vi "TIO Stream Write.vi"(6 "Routing":string, 7 "error in (no error)":errorcluster, 8 "Type":T1(ring)=enum."RPC Request", 9 "Payload":string, 10 "TS Connection":T2={"Type"=enum."TCP", "Serial"="serial:///dev/cu.usbserial-00000", "TCP"=refnum, "Timeout"=500}) -> (0 "error out":errorcluster, 3 "TS Connection":T2={"Type"=enum."TCP", "Serial"="serial:///dev/cu.usbserial-00000", "TCP"=refnum, "Timeout"=500})   [LabVIEW 2016]
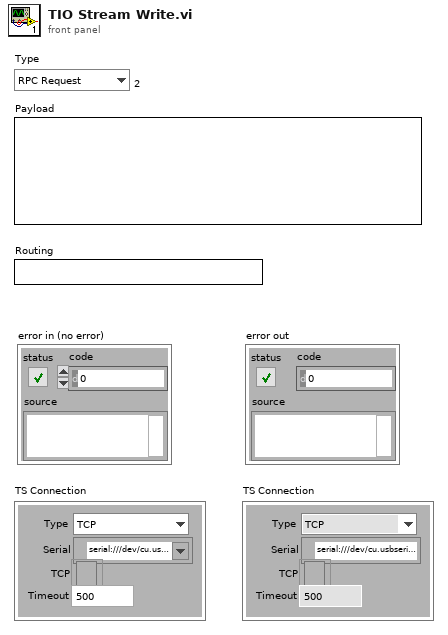
[diagram p1: front panel]
types:
  T1 = enum8{"Invalid", "Log", "RPC Request", "RPC Reply", "RPC Error", "Stream Description", "User"}
  T2 = cluster{"Type":enum16{"TCP", "Serial"}, "Serial":refnum<visa-resource-name>, "TCP":refnum<k5>, "Timeout":u32}
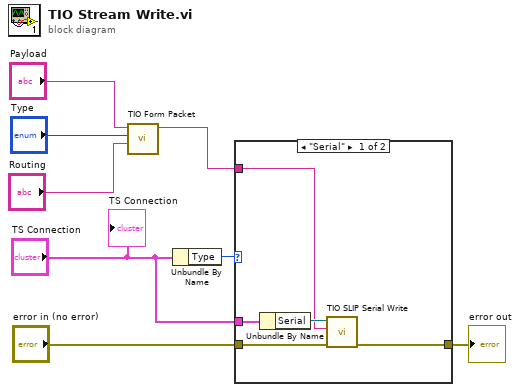
[diagram p0: block diagram]
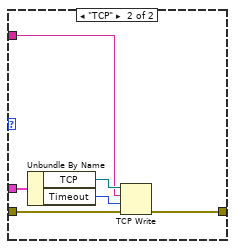
[diagram p2: hidden frame]
diagram:
  n1 = call "TIO Form Packet.vi"("Routing"="Routing", "Type"="Type", "Payload"="Payload") -> ("String out"=w3:string)  [unwired: 8 in]
  n2 = Unbundle By Name("TS Connection") -> ("Type"=w8:enum16{"TCP", "Serial"})
  n3 = case shown="\"Serial\"" w8 {
    tunnel: w3 -> [w9 w14]
    tunnel: "TS Connection" -> [w13 w19]
    tunnel: "error in (no error)" -> [w11 w17]
    tunnel: [w10 w15] -> w6
    frame "Serial" {
      n4 = Unbundle By Name(w13) -> ("Serial"=w12:refnum<visa-resource-name>)
      n5 = call "TIO SLIP Serial Write.vi"("error in (no error)"=w11, "Data"=w9, "VISA Refnum in"=w12) -> ("error out"=w10:errorcluster)  [unwired: 8 in]
    }
    frame "TCP" {
      n6 = Unbundle By Name(w19) -> ("TCP"=w18:refnum<k5>, "Timeout"=w16:u32)
      n7 = TCP Write(connection ID=w18, data in=w14, error in (no error)=w17, 9:w16) -> (error out=w15:errorcluster)  [unwired: 2 out]
    }
  }
  "error out" <- w6
  "TS Connection" <- "TS Connection"
